vi "Rotate Arms (David Guan).vi"(11 "Open?":bool) -> ()   [LabVIEW 2014]
uses:
  <vilib>/Rock Robotics/WPI/Solenoid/Deprecated/WPI_SolenoidSetBool.vi
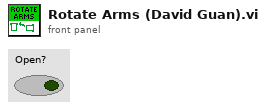
[diagram p1: front panel]
types:
  T1 = typedef "WPI_SolenoidDevRef.ctl" = cluster{"DevStatus":errorcluster, "Pneumatics Control Module":u8, "Forward Solenoid Channel":T2, "Reverse Solenoid Channel":T2}
  T2 = typedef "WPI_SolenoidChannel.ctl" = enum8{"Solenoid 0", "Solenoid 1", "Solenoid 2", "Solenoid 3", "Solenoid 4", "Solenoid 5", "Solenoid 6", "Solenoid 7", "Invalid"}
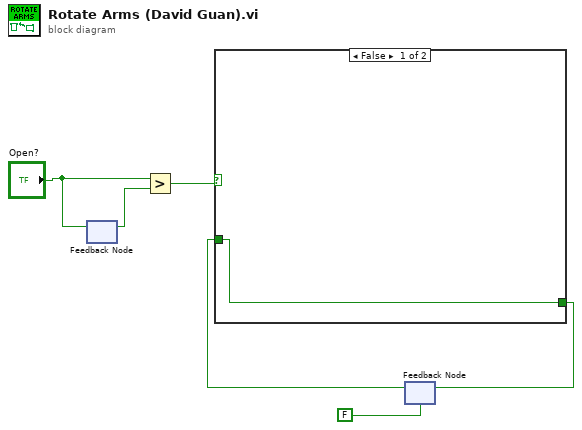
[diagram p0: block diagram]
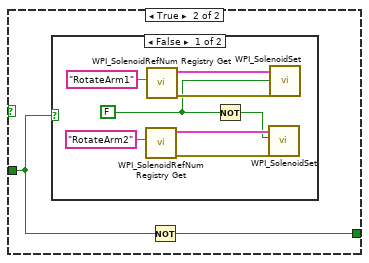
[diagram p2: hidden frame]
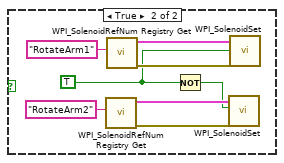
[diagram p3: hidden frame]
diagram:
  n1 = feedback-in #1("Open?") -> ()
  n2 = feedback #1() -> (w5:bool)  [unwired: 1 in]
  n3 = Greater?(x="Open?", y=w5) -> (0:w4:bool)
  n4 = feedback #2(FALSE) -> (w2:bool)
  n5 = case shown="False" w4 {
    tunnel: w2 -> [w7 w9]
    tunnel: [w7 w8] -> w1
    frame False {
    }
    frame True {
      n6 = case shown="False" w9 {
        frame False {
          w10 = FALSE
          n7 = call <vilib>:"WPI_SolenoidRefNum Registry Get.vi"("refnum name"="RotateArm2") -> ("error out"=w13:errorcluster, "SolenoidDevRef"=w14:T1)  [unwired: 9 in]
          n8 = call <vilib>:"WPI_SolenoidRefNum Registry Get.vi"("refnum name"="RotateArm1") -> ("error out"=w16:errorcluster, "SolenoidDevRef"=w17:T1)  [unwired: 9 in]
          n9 = Not(x=w10) -> (.not. x?=w11:bool)
          n10 = call-poly <vilib>:"WPI_SolenoidSet.vi"("error in (no error)"=w13, "Value"=w11, "SolenoidDevRef"=w14) -> ()  [unwired: 7 in, 2 out]
          n11 = call-poly <vilib>:"WPI_SolenoidSet.vi"("error in (no error)"=w16, "Value"=w10, "SolenoidDevRef"=w17) -> ()  [unwired: 7 in, 2 out]
        }
        frame True {
          w18 = TRUE
          n12 = call <vilib>:"WPI_SolenoidRefNum Registry Get.vi"("refnum name"="RotateArm2") -> ("error out"=w21:errorcluster, "SolenoidDevRef"=w22:T1)  [unwired: 9 in]
          n13 = call <vilib>:"WPI_SolenoidRefNum Registry Get.vi"("refnum name"="RotateArm1") -> ("error out"=w24:errorcluster, "SolenoidDevRef"=w25:T1)  [unwired: 9 in]
          n14 = Not(x=w18) -> (.not. x?=w19:bool)
          n15 = call-poly <vilib>:"WPI_SolenoidSet.vi"("error in (no error)"=w21, "Value"=w19, "SolenoidDevRef"=w22) -> ()  [unwired: 7 in, 2 out]
          n16 = call-poly <vilib>:"WPI_SolenoidSet.vi"("error in (no error)"=w24, "Value"=w18, "SolenoidDevRef"=w25) -> ()  [unwired: 7 in, 2 out]
        }
      }
      n17 = Not(x=w9) -> (.not. x?=w8:bool)
    }
  }
  n18 = feedback-in #2(w1) -> ()
